vi "Filter Binary To Text.vi"(11 "Raw input":u8[](array[numeric])) -> (3 "Filtered output":u8[](array[numeric]))   [LabVIEW 2017, in "SLSC Switch Scripting.lvlib"]
uses:
  SLSC Switch Scripting.lvlib
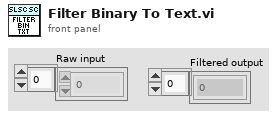
[diagram p1: front panel]
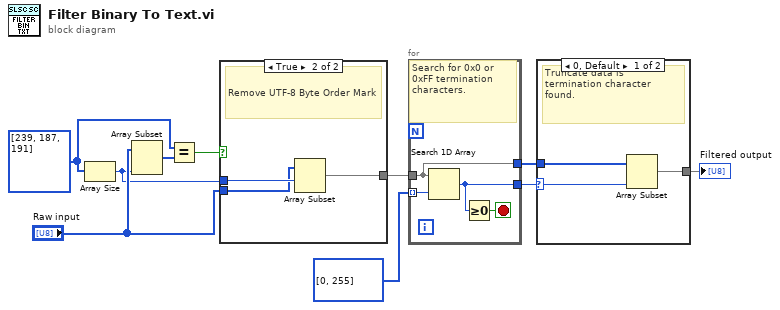
[diagram p0: block diagram]
diagram:
  w5 = u8[] [239, 187, 191]
  n1 = Array Size(array=w5) -> (size(s)=w7:i32)
  n2 = Array Subset(array="Raw input", length=w7) -> (w4:u8[])  [unwired: 1 in]
  n3 = Equal?(x=w5, y=w4) -> (x = y?=w6:bool)
  n4 = case shown="True" w6 {
    tunnel: w7 -> [_ w14]
    tunnel: "Raw input" -> [w11 w13]
    tunnel: [w11 w12] -> w10
    frame False {
      # "No UTF-8 Byte Order Mark"
    }
    frame True {
      # "Remove UTF-8 Byte Order Mark"
      n5 = Array Subset(array=w13, index=w14) -> (w12:u8[])  [unwired: 1 in]
    }
  }
  n6 = for {
    tunnel: w10 -> [w15]
    tunnel: [w17] -> w9
    tunnel: u8[] [0, 255] -> [w18] mode=indexing
    tunnel: [w15] -> w2
    stop <- w16 stop-if-true
    # "Search for 0x0 or 0xFF termination characters."
    n7 = Search 1D Array(1D array=w15, element=w18) -> (index of element=w17:i32)  [unwired: 1 in]
    n8 = Greater Or Equal To 0?(x=w17) -> (x >= 0?=w16:bool)
  }
  n9 = case shown="0, Default" w9 {
    selector: w9 -> [w19 _]
    tunnel: w2 -> [w21 w22]
    tunnel: [w20 w22] -> w1
    frame 0, Default {
      # "Truncate data is termination character found."
      n10 = Array Subset(array=w21, length=w19) -> (w20:u8[])  [unwired: 1 in]
    }
    frame -1 {
      # "No NUL character."
    }
  }
  "Filtered output" <- w1
